vi "SkidpadRetryRoll.vi"(11 "InternalData":T1={"CurrentRecordIndicator"={"Lab2"="", "Lab4"="", "TotalLabTime"="", "CurrentEntry"="", "CurrentSchool"="", "Flag"=bytes[0], "Message"="", "LapProgress"={"Lap-1"=FALSE, "Lap-2"=FALSE, "Lap-3"=FALSE, "Lap-4"=FALSE}, "EventCount"={"Attempt-1"=FALSE, "Attempt-2"=FALSE, "Attempt-3"=FALSE, "Attempt-4"=FALSE}}, "BestRecordIndicator"={"BestTime"="", "BestEntry"="", "BestUniv"=""}, "FlagData"={"GreenFlag"=bytes[0], "BlueFlag"=bytes[0], "RedFlag"=bytes[0], "CheckFlag"=bytes[0]}, "InternalTimmer"={"1LapRefTime"=0, "1LapTime"=0, "2LapRefTime"=0, "2LapTime"=0, "3LapRefTime"=0, "3LapTime"=0, "4LapRefTime"=0, "4LapTime"=0, "TotalLabTime"=0}, "StateValue"=enum."Initial", "EventProgressData"=[], "Ready"=FALSE, "Retry"=FALSE, "DNF"=FALSE, "NextEntry"=FALSE, "ProgramStop"=FALSE}) -> (3 "InternalData 2":T1={"CurrentRecordIndicator"={"Lab2"="", "Lab4"="", "TotalLabTime"="", "CurrentEntry"="", "CurrentSchool"="", "Flag"=bytes[0], "Message"="", "LapProgress"={"Lap-1"=FALSE, "Lap-2"=FALSE, "Lap-3"=FALSE, "Lap-4"=FALSE}, "EventCount"={"Attempt-1"=FALSE, "Attempt-2"=FALSE, "Attempt-3"=FALSE, "Attempt-4"=FALSE}}, "BestRecordIndicator"={"BestTime"="", "BestEntry"="", "BestUniv"=""}, "FlagData"={"GreenFlag"=bytes[0], "BlueFlag"=bytes[0], "RedFlag"=bytes[0], "CheckFlag"=bytes[0]}, "InternalTimmer"={"1LapRefTime"=0, "1LapTime"=0, "2LapRefTime"=0, "2LapTime"=0, "3LapRefTime"=0, "3LapTime"=0, "4LapRefTime"=0, "4LapTime"=0, "TotalLabTime"=0}, "StateValue"=enum."Initial", "EventProgressData"=[], "Ready"=FALSE, "Retry"=FALSE, "DNF"=FALSE, "NextEntry"=FALSE, "ProgramStop"=FALSE})   [LabVIEW 2020]
uses:
  Control/SkidpadInternalVariable.ctl
  Control/SkidpadCurrentRecordIndicator.ctl
  Control/SkidpadBestRecordIndicator.ctl
  CommonControl/Flag.ctl
  Control/SkidpadInternalTimmer.ctl
  Control/SkidpadState.ctl
panel:
  # "Lap2 :"
  # "Lap4 :"
  # "Total :"
  # "Entry :"
  # "#1"
  # "#2"
  # "#3"
  # "#4"
  # "Univ. :"
  # "Lap2 :"
  # "Lap4 :"
  # "Total :"
  # "Entry :"
  # "#1"
  # "#2"
  # "#3"
  # "#4"
  # "Univ. :"
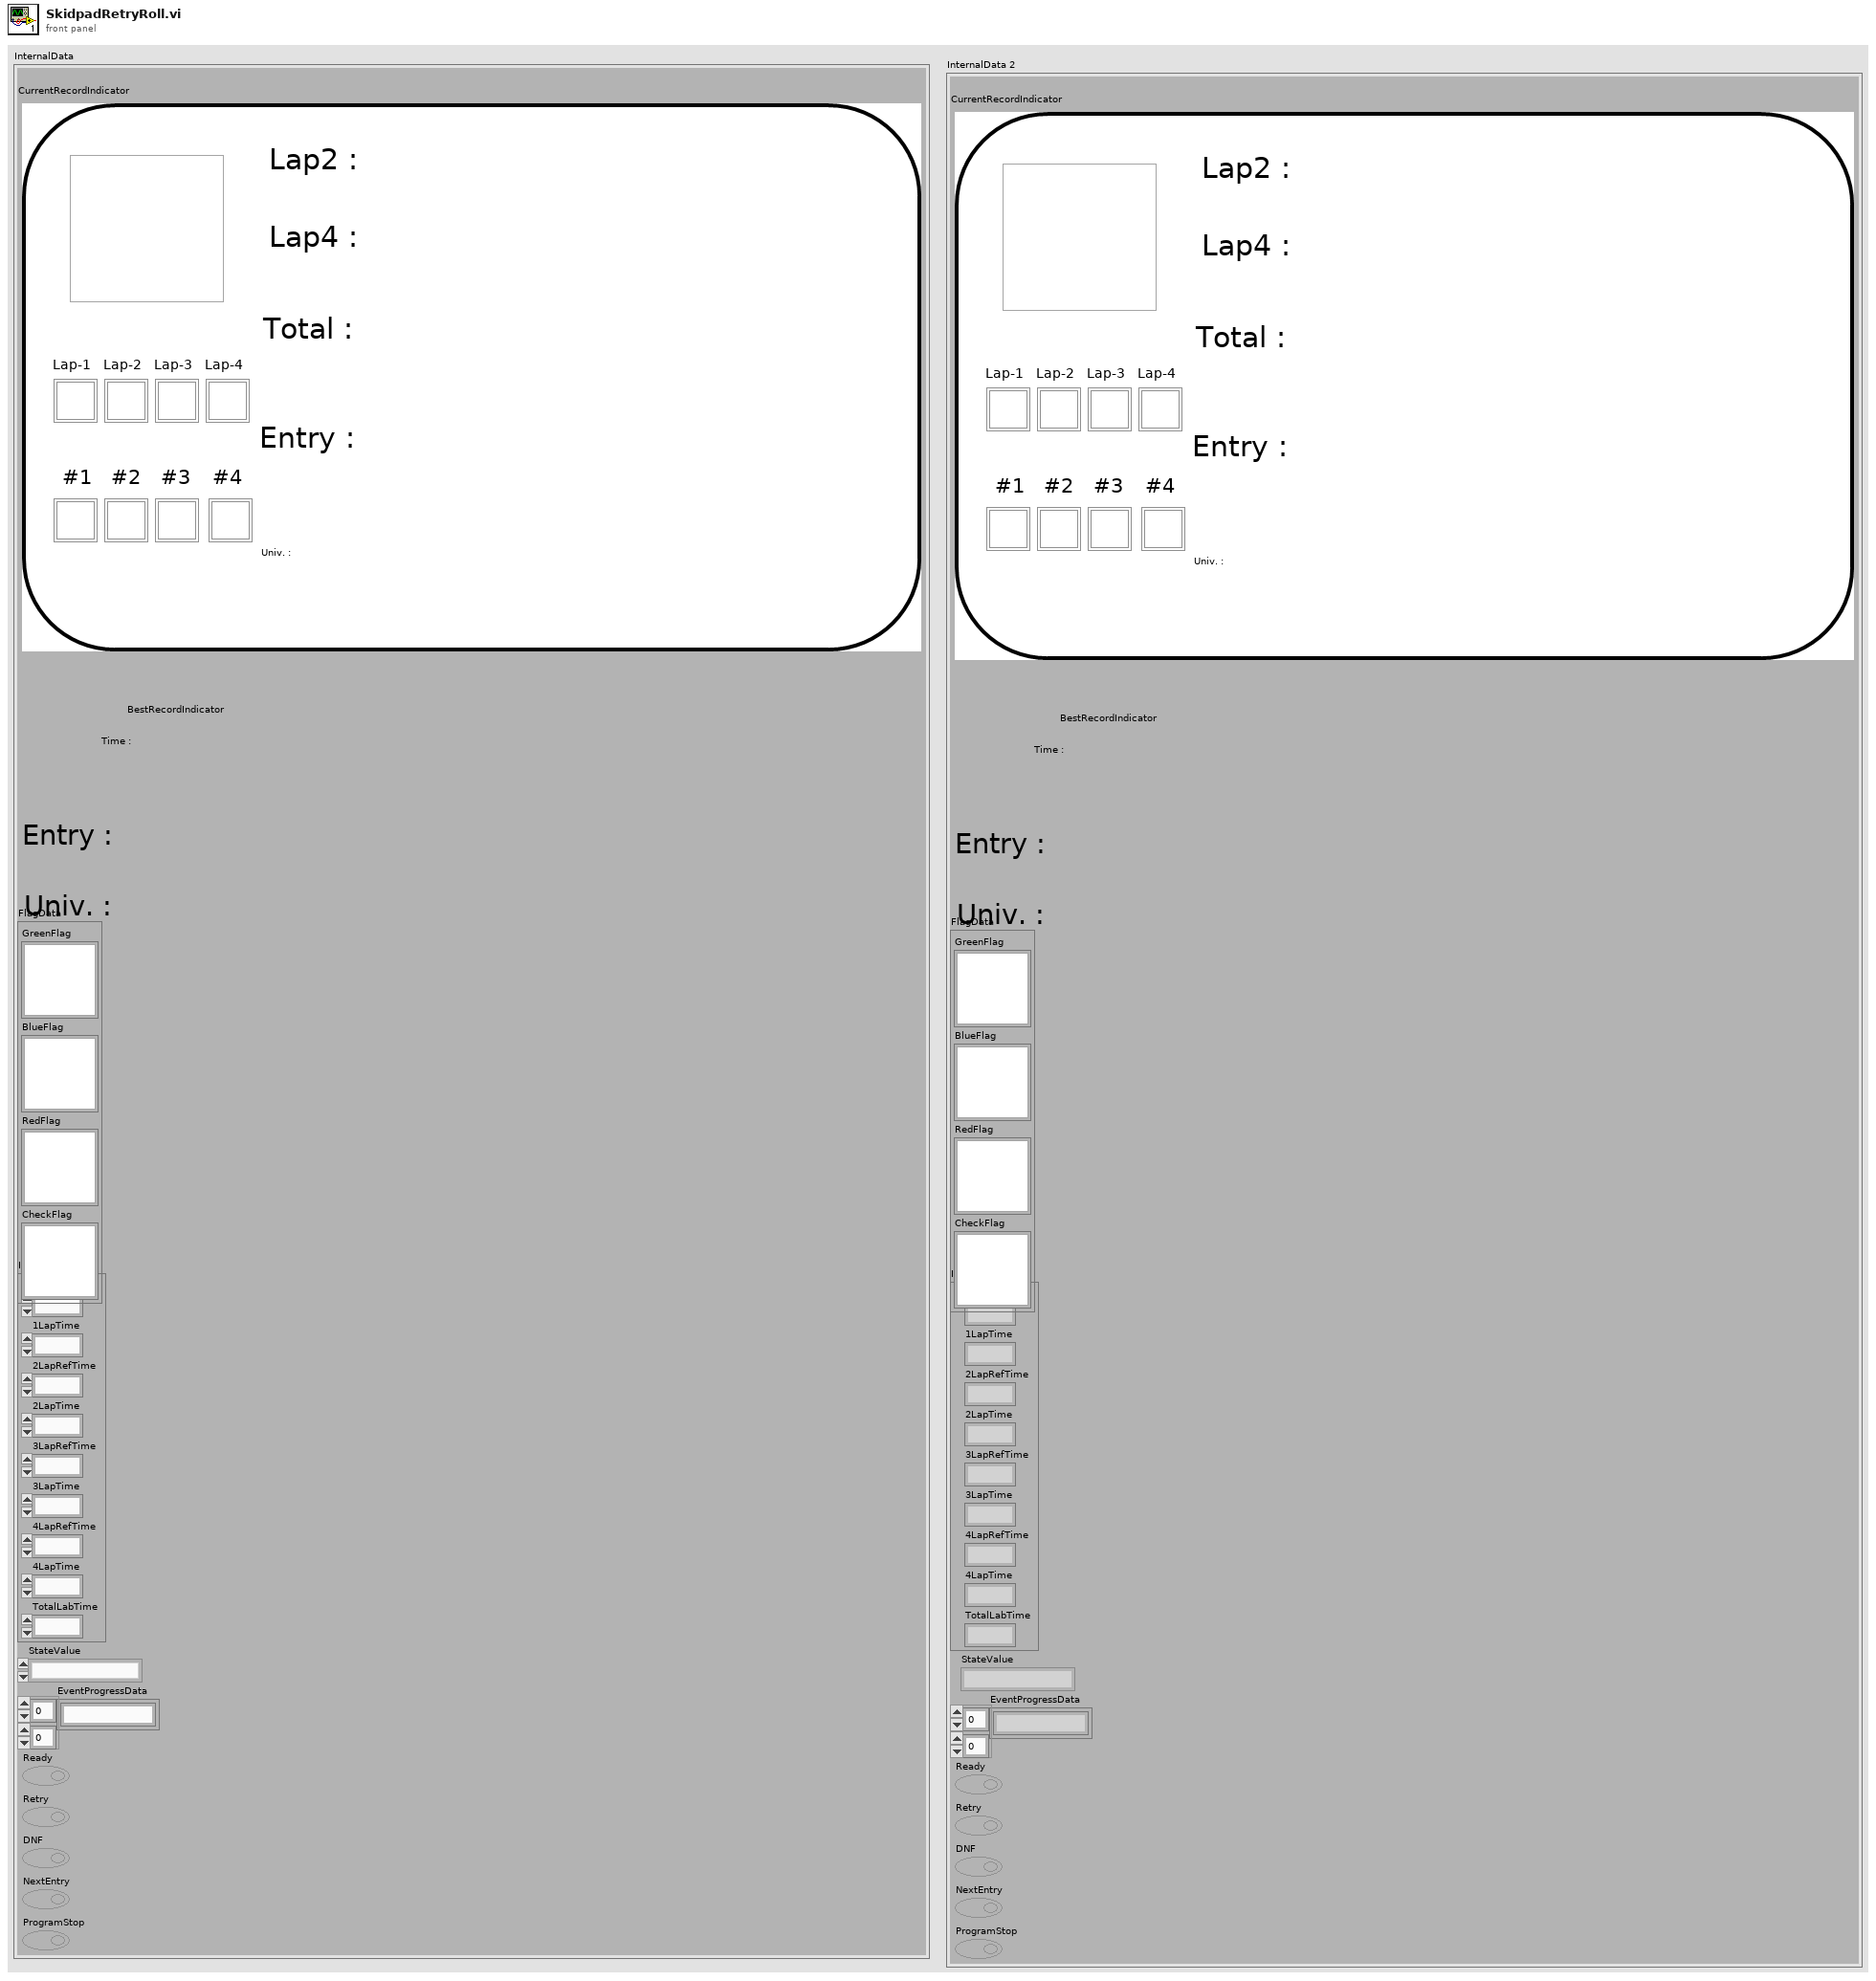
[diagram p1: front panel]
types:
  T1 = typedef "SkidpadInternalVariable.ctl" = cluster{"CurrentRecordIndicator":T2, "BestRecordIndicator":T3, "FlagData":T4, "InternalTimmer":T5, "StateValue":T6, "EventProgressData":string[][], "Ready":bool, "Retry":bool, "DNF":bool, "NextEntry":bool, "ProgramStop":bool}
  T2 = typedef "SkidpadCurrentRecordIndicator.ctl" = cluster{"Lab2":string, "Lab4":string, "TotalLabTime":string, "CurrentEntry":string, "CurrentSchool":string, "Flag":picture, "Message":string, "LapProgress":cluster{"Lap-1":bool, "Lap-2":bool, "Lap-3":bool, "Lap-4":bool}, "EventCount":cluster{"Attempt-1":bool, "Attempt-2":bool, "Attempt-3":bool, "Attempt-4":bool}}
  T3 = typedef "SkidpadBestRecordIndicator.ctl" = cluster{"BestTime":string, "BestEntry":string, "BestUniv":string}
  T4 = typedef "Flag.ctl" = cluster{"GreenFlag":picture, "BlueFlag":picture, "RedFlag":picture, "CheckFlag":picture}
  T5 = typedef "SkidpadInternalTimmer.ctl" = cluster{"1LapRefTime":i64, "1LapTime":i64, "2LapRefTime":i64, "2LapTime":i64, "3LapRefTime":i64, "3LapTime":i64, "4LapRefTime":i64, "4LapTime":i64, "TotalLabTime":i64}
  T6 = typedef "SkidpadState.ctl" = enum16{"Initial", "InputInfomation", "Ready", "1lap", "2lap", "3lap", "4lap", "FinshRunning", "LogRecord", "HardwareRelease", "WaittingforNext", "ProgramStop"}
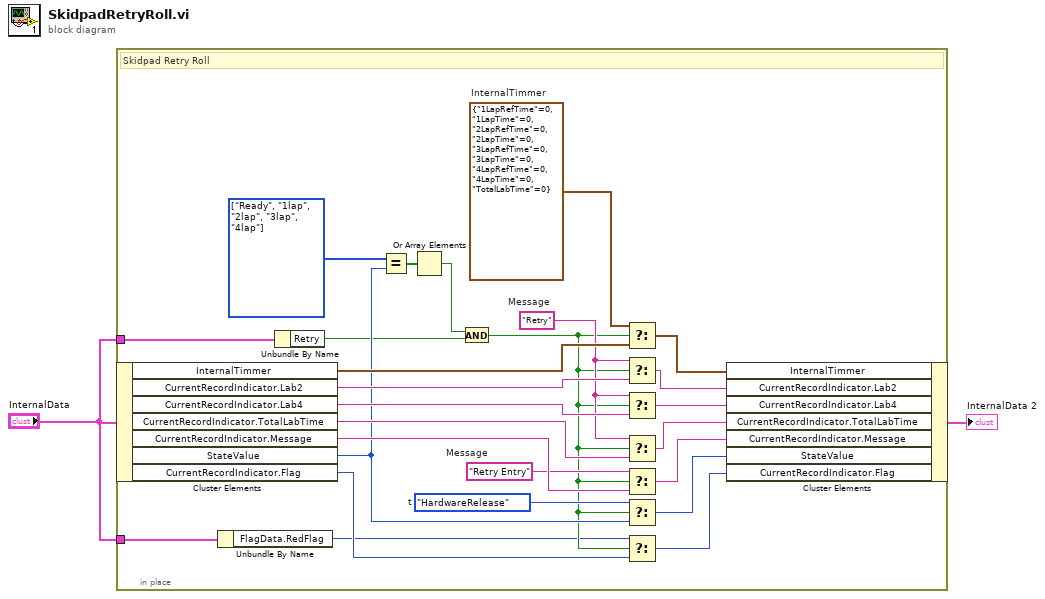
[diagram p0: block diagram]
diagram:
  n1 = in-place {
    in-place-border: "InternalData" -> [w9]
    in-place-border: "InternalData" -> [w4]
    w10 = "Retry"  # Message
    w13 = T6[] [enum."Ready", enum."1lap", enum."2lap", enum."3lap", enum."4lap"] items=["Initial", "InputInfomation", "Ready", "1lap", "2lap", "3lap", "4lap", "FinshRunning", "LogRecord", "HardwareRelease", "WaittingforNext", "ProgramStop"]
    w15 = SkidpadState."HardwareRelease"  # t
    w18 = "Retry Entry"  # Message
    w27 = T5 {"1LapRefTime"=0, "1LapTime"=0, "2LapRefTime"=0, "2LapTime"=0, "3LapRefTime"=0, "3LapTime"=0, "4LapRefTime"=0, "4LapTime"=0, "TotalLabTime"=0}  # InternalTimmer
    # "Skidpad Retry Roll"
    n2 = in-place-cluster #1("InternalData") -> ("InternalTimmer"=w28:T5, "CurrentRecordIndicator.Lab2"=w25:string, "CurrentRecordIndicator.Lab4"=w23:string, "CurrentRecordIndicator.TotalLabTime"=w21:string, "CurrentRecordIndicator.Message"=w19:string, "StateValue"=w14:T6, "CurrentRecordIndicator.Flag"=w7:picture)
    n3 = Unbundle By Name(w9) -> ("FlagData.RedFlag"=w6:picture)
    n4 = Unbundle By Name(w4) -> ("Retry"=w3:bool)
    n5 = Equal?(x=w13, y=w14) -> (x = y?=w12:bool[])
    n6 = Or Array Elements(Boolean array=w12) -> (logical OR=w11:bool)
    n7 = And(x=w11, y=w3) -> (x .and. y?=w8:bool)
    n8 = Select(t=w27, s=w8, f=w28) -> (s? t:f=w26:T5)
    n9 = Select(t=w10, s=w8, f=w25) -> (s? t:f=w24:string)
    n10 = Select(t=w10, s=w8, f=w23) -> (s? t:f=w22:string)
    n11 = Select(t=w10, s=w8, f=w21) -> (s? t:f=w20:string)
    n12 = Select(t=w18, s=w8, f=w19) -> (s? t:f=w17:string)
    n13 = Select(t=w15, s=w8, f=w14) -> (s? t:f=w16:T6)
    n14 = Select(t=w6, s=w8, f=w7) -> (s? t:f=w5:picture)
    n15 = in-place-cluster #1("InternalTimmer"=w26, "CurrentRecordIndicator.Lab2"=w24, "CurrentRecordIndicator.Lab4"=w22, "CurrentRecordIndicator.TotalLabTime"=w20, "CurrentRecordIndicator.Message"=w17, "StateValue"=w16, "CurrentRecordIndicator.Flag"=w5) -> (→"InternalData 2":T1)
  }
